vi "Log Channels.vi"(8 "monitoring channel offsets":u64[](array[numeric]), 9 "monitoring channels refs":T1[](array[typedef]) format="%.0x", 10 "data channel offsets":u64[](array[numeric]), 11 "data channels refs":T1[](array[typedef]) format="%.0x") -> ()   [LabVIEW 2017, in "DSF Engine.lvlib" / "VeriStand DSF.lvclass"]
uses:
  VeriStand DSF.lvclass
  <vilib>/NI Veristand/Custom Device API/Custom Device Item Ref.ctl
  <vilib>/NI Veristand/Custom Device API/Custom Device API.lvlib
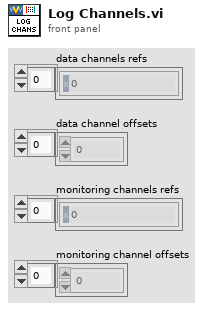
[diagram p1: front panel]
types:
  T1 = typedef "Custom Device API.lvlib/Custom Device Item Ref.ctl" = u64
  T2 = enum16{"open", "replace", "create", "open or create", "replace or create", "replace or create with confirmation"}
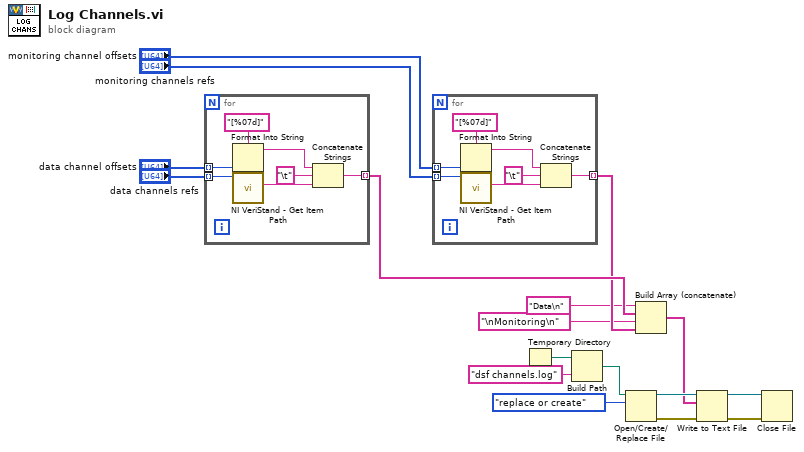
[diagram p0: block diagram]
diagram:
  n1 = for {
    tunnel: [w22] -> w17 mode=indexing
    tunnel: "data channel offsets" -> [w18] mode=indexing
    tunnel: "data channels refs" -> [w21] mode=indexing
    n2 = Format Into String(format string="[%07d]", w18) -> (resulting string=w19:string)  [unwired: 2 in, 1 out]
    n3 = call <vilib>:"NI VeriStand - Get Item Path.vi"("Item Ref in"=w21) -> ("Path"=w23:string)  [unwired: 7 in, 3 out]
    n4 = Concatenate Strings(w19, "\t" ("string"), w23) -> (w22:string)
  }
  n5 = for {
    tunnel: [w28] -> w12 mode=indexing
    tunnel: "monitoring channel offsets" -> [w25] mode=indexing
    tunnel: "monitoring channels refs" -> [w30] mode=indexing
    n6 = Format Into String(format string="[%07d]", w25) -> (resulting string=w26:string)  [unwired: 2 in, 1 out]
    n7 = call <vilib>:"NI VeriStand - Get Item Path.vi"("Item Ref in"=w30) -> ("Path"=w29:string)  [unwired: 7 in, 3 out]
    n8 = Concatenate Strings(w26, "\t" ("string"), w29) -> (w28:string)
  }
  n9 = Temporary Directory() -> (w10:path)
  n10 = Build Path(base path=w10, name or relative path="dsf channels.log") -> (appended path=w8:path)
  n11 = Open/Create/Replace File(file path (use dialog)=w8, operation (0:open)=T2."replace or create") -> (refnum out=w7:refnum<file>, error out=w6:errorcluster)  [unwired: 4 in, 1 out]
  n12 = Build Array (concatenate)("Data\n", w17, "\nMonitoring\n", w12) -> (w1:string[])
  n13 = Write to Text File(file (use dialog)=w7, text=w1, error in=w6) -> (refnum out=w4:refnum<file>, error out=w5:errorcluster)  [unwired: 1 in, 1 out]
  n14 = Close File(refnum=w4, error in=w5) -> ()  [unwired: 2 out]
